vi "Configure Marker Peak Search.vi"(0 "VISA resource name":refnum<visa-resource-name>, 1 "Enable Continuous Peak Search (T: Enable)":bool=TRUE, 5 "Active Marker (1: Marker 1)":i32(ring)=1 items=["Marker 1"=1, "Marker 2"=2, "Marker 3"=3, "Marker 4"=4, "Marker 5"=5, "Marker 6"=6], 7 "Marker Search (0: Maximum)":i32(ring) items=["Maximum", "Next Peak", "Next Peak Left", "Next Peak Right", "Peak to Peak"], 9 "Peak Search (0: Maximum)":i32(ring) items=["Maximum", "Minimum"], 11 "error in (no error)":errorcluster, 12 "Peak Excursion (0)":dbl, 13 "Peak Threshold (-140 dBm)":dbl=-140.0) -> (4 "VISA resource name out":refnum<visa-resource-name>, 15 "error out":errorcluster)   [LabVIEW 2022 SP3, in "Agilent N934X Series.lvlib"]
doc: "Configures the marker peak search settings on the spectrum analyzer."
uses:
  <instrlib>/Agilent N934X Series/Agilent N934X Series.lvlib
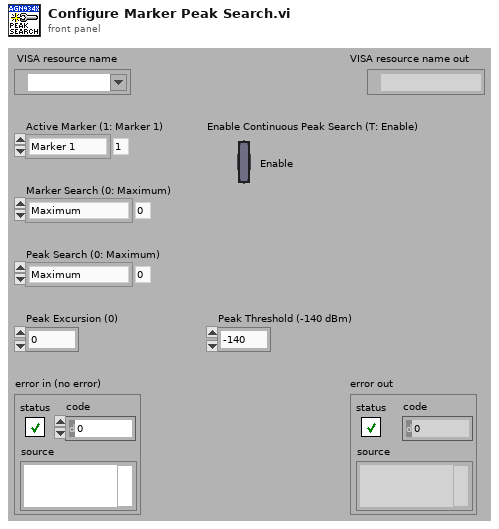
[diagram p1: front panel]
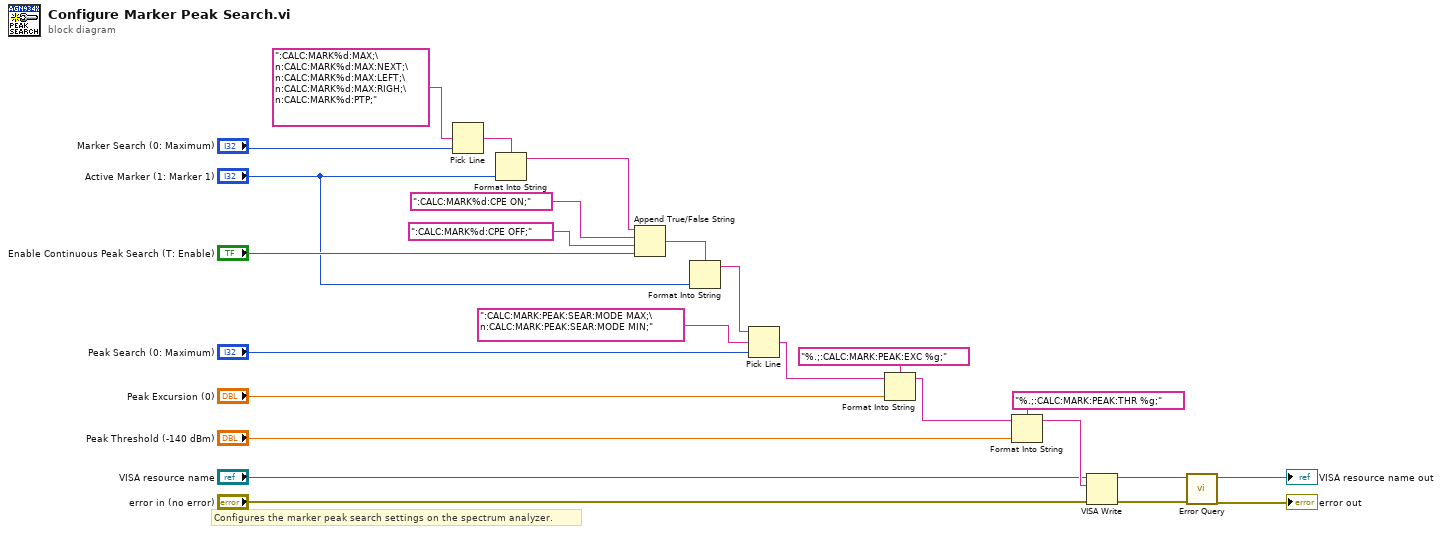
[diagram p0: block diagram]
diagram:
  # "Configures the marker peak search settings on the spectrum analyzer."
  n1 = Pick Line(multi-line string=":CALC:MARK%d:MAX;\n:CALC:MARK%d:MAX:NEXT;\n:CALC:MARK%d:MAX:LEFT;\n:CALC:MARK%d:MAX:RIGH;\n:CALC:MARK%d:PTP;", line index="Marker Search (0: Maximum)") -> (output string=w12:string)  [unwired: 1 in]
  n2 = Format Into String(format string=w12, "Active Marker (1: Marker 1)") -> (resulting string=w5:string)  [unwired: 2 in, 1 out]
  n3 = Append True/False String(1:"Enable Continuous Peak Search (T: Enable)", 2:":CALC:MARK%d:CPE OFF;", 3:":CALC:MARK%d:CPE ON;", 4:w5) -> (0:w3:string)
  n4 = Format Into String(format string=w3, "Active Marker (1: Marker 1)") -> (resulting string=w2:string)  [unwired: 2 in, 1 out]
  n5 = Pick Line(string ("")=w2, multi-line string=":CALC:MARK:PEAK:SEAR:MODE MAX;\n:CALC:MARK:PEAK:SEAR:MODE MIN;", line index="Peak Search (0: Maximum)") -> (output string=w8:string)
  n6 = Format Into String(format string="%.;:CALC:MARK:PEAK:EXC %g;", initial string=w8, "Peak Excursion (0)") -> (resulting string=w4:string)  [unwired: 1 in, 1 out]
  n7 = Format Into String(format string="%.;:CALC:MARK:PEAK:THR %g;", initial string=w4, "Peak Threshold (-140 dBm)") -> (resulting string=w21:string)  [unwired: 1 in, 1 out]
  n8 = VISA Write(VISA resource name="VISA resource name", write buffer=w21, error in (no error)="error in (no error)") -> (VISA resource name out=w18:refnum<visa-resource-name>, error out=w17:errorcluster)  [unwired: 1 out]
  n9 = call <instrlib>:"Error Query.vi"("error in (no error)"=w17, "VISA resource name"=w18) -> ("error out"=→"error out":errorcluster, "VISA resource name out"=→"VISA resource name out":refnum<visa-resource-name>)  [unwired: 6 in, 2 out]
